vi "Read All Settings IDs.vi"(8 "error in (no error)":errorcluster, 11 "dsf refnum":T1) -> (0 "error out":errorcluster, 1 "Setting IDs":string[](array[string]), 3 "dsf refnum out":T1)   [LabVIEW 2017, in "DSF Configuration API.lvlib"]
doc: "Gets the names of all sections from the configuration data identified by <B>dsf refnum</B>."
uses:
  DSF Configuration API.lvlib
  Controls/DSF Config Data RefNum.ctl
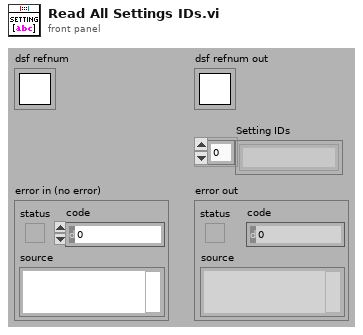
[diagram p1: front panel]
types:
  T1 = typedef "DSF Configuration API.lvlib/DSF Config Data RefNum.ctl" = refnum<k1>
  T2 = typedef "DSF Configuration API.lvlib/DSF Configuration Reference.ctl" = refnum<data-value>
  T3 = typedef "DSF Configuration API.lvlib/Internal.DSF Configuration.ctl" = cluster{"dsfversion":T4, "version":T4, "plugins":T5[], "groups":T8[], "transfers":T10[], "channels":T12[], "settings":T14[]}
  T4 = typedef "DSF Configuration API.lvlib/DSF Version Info.ctl" = cluster{"major":u32, "minor":u32, "fix":u32, "build":string}
  T5 = typedef "DSF Configuration API.lvlib/Internal.DSF Plugin with ID.ctl" = cluster{"id":string, "values":T6}
  T6 = typedef "DSF Configuration API.lvlib/Internal.DSF Plugin Info.ctl" = cluster{"type":string, "timing":T7, "group ids":string[], "settings id":string}
  T7 = typedef "DSF Configuration API.lvlib/DSF Timing Info.ctl" = cluster{"priority":u64, "decimation":u64, "offset":u64}
  T8 = typedef "DSF Configuration API.lvlib/Internal.DSF Group with ID.ctl" = cluster{"id":string, "values":T9}
  T9 = typedef "DSF Configuration API.lvlib/Internal.DSF Group Info.ctl" = cluster{"direction":i32, "timing":T7, "transfer ids":string[], "settings id":string}
  T10 = typedef "DSF Configuration API.lvlib/Internal.DSF Transfer with ID.ctl" = cluster{"id":string, "values":T11}
  T11 = typedef "DSF Configuration API.lvlib/Internal.DSF Transfer Info.ctl" = cluster{"byte order":i32, "channel ids":string[], "settings id":string}
  T12 = typedef "DSF Configuration API.lvlib/Internal.DSF Channel with ID.ctl" = cluster{"id":string, "values":T13}
  T13 = typedef "DSF Configuration API.lvlib/Internal.DSF Channel Info.ctl" = cluster{"count":u64, "buffer offset":u64, "data type":i32, "settings id":string}
  T14 = typedef "DSF Configuration API.lvlib/Internal.DSF Settings with ID.ctl" = cluster{"id":string, "values":T15}
  T15 = typedef "DSF Configuration API.lvlib/Internal.DSF Settings Info.ctl" = cluster{"key":string, "value":string}[]
  T16 = cluster{"dsf configuration":T3, "path":path, "dirty":bool}
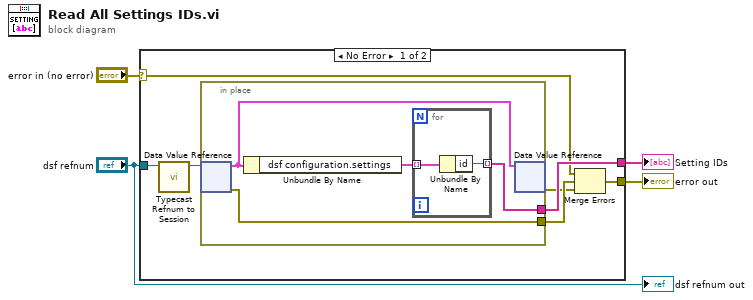
[diagram p0: block diagram]
diagram:
  n1 = case shown="No Error" "error in (no error)" {
    selector: "error in (no error)" -> [w9 w18]
    tunnel: [w11 _] -> w2
    tunnel: [w7 w18] -> w3
    tunnel: "dsf refnum" -> [w10 _]
    frame No Error {
      n2 = call "Typecast Refnum to Session.vi"("dsf refnum in"=w10) -> ("DSF Configuration Session out"=w8:T2)  [unwired: 10 in]
      n3 = in-place {
        in-place-border: [w15] -> w11
        in-place-border: [w12] -> w6
        n4 = in-place-dvr #1(w8) -> (w13:T16, w12:errorcluster)
        n5 = Unbundle By Name(w13) -> ("dsf configuration.settings"=w14:T14[])
        n6 = for {
          tunnel: w14 -> [w16] mode=indexing
          tunnel: [w17] -> w15 mode=indexing
          n7 = Unbundle By Name(w16) -> ("id"=w17:string)
        }
        n8 = in-place-dvr #1(w13) -> (w5:errorcluster)  [unwired: 1 out]
      }
      n9 = Merge Errors(w9, w6, w5) -> (w7:errorcluster)
    }
    frame Error {
    }
  }
  "error out" <- w3
  "Setting IDs" <- w2
  "dsf refnum out" <- "dsf refnum"
